vi "TLS Client.vi"() -> ()   [LabVIEW 2020, in "Test.lvlib"]
uses:
  Test.lvlib
  TCP Comms/TinyTCP.lvlib
  TCP Comms/Cert Chain.ctl
  TCP Comms/Client TLS Config.ctl
  346ab590-12ca-473f-8f0a-edbb0b931e8c.vi
  3b2e32dd-1c02-490c-a519-554a5f01b085.vi
  Server Data.ctl
  TCP Comms/State.ctl
  Client Data.ctl
panel:
  out "Error":errorcluster
  out "Server Data":T1
  in  "Client Data":T2 {"Slide" scale=0.0..10.0}
  in  "Close":bool
  in  "Open":bool
  out "Client State":T3
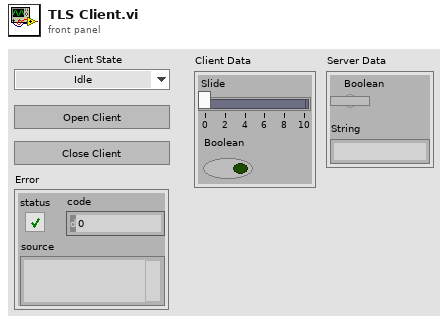
[diagram p1: front panel]
types:
  T1 = typedef "Test.lvlib/Server Data.ctl" = cluster{"Boolean":bool, "String":string}
  T2 = typedef "Test.lvlib/Client Data.ctl" = cluster{"Slide":dbl, "Boolean":bool}
  T3 = typedef "TinyTCP.lvlib/State.ctl" = enum16{"Idle", "Starting", "Connecting", "Connected", "Disconnecting", "Stopped"}
  T4 = typedef "TinyTCP.lvlib/Cert Chain.ctl" = cluster{"Path":path, "Format":enum32{"X.509 (PEM)"}}
  T5 = typedef "TinyTCP.lvlib/Client TLS Config.ctl" = cluster{"Use OS Certificates":bool, "Cert Chains":T4[], "Server Cert Name":string}
  T6 = typedef "TinyTCP.lvlib/Instance.ctl" = refnum<data-value>
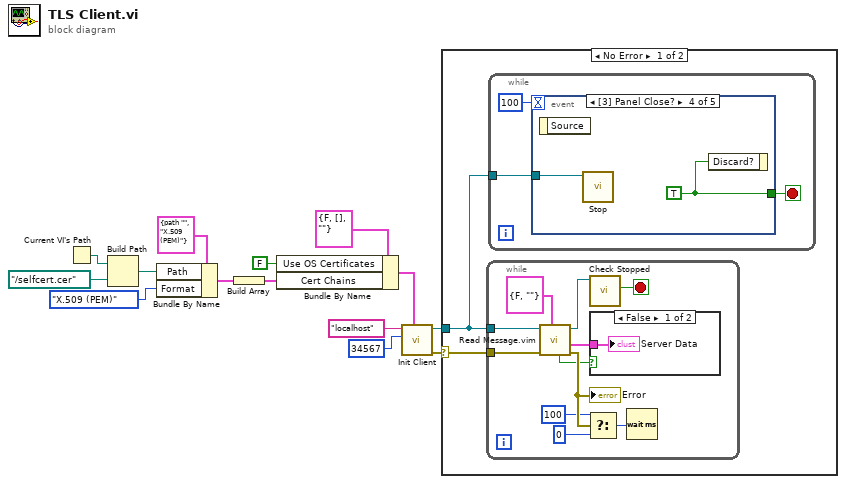
[diagram p0: block diagram]
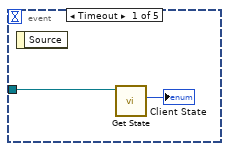
[diagram p3: hidden frame]
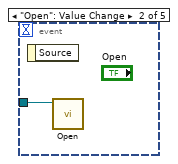
[diagram p4: hidden frame]
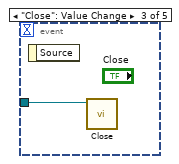
[diagram p5: hidden frame]
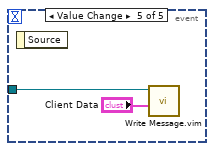
[diagram p6: hidden frame]
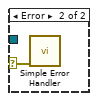
[diagram p7: hidden frame]
diagram:
  n1 = Current VI's Path() -> (path=w10:path)
  n2 = Build Path(base path=w10, name or relative path=path "../selfcert.cer") -> (appended path=w8:path)
  n3 = Bundle By Name(cluster=T4 {"Path"=path "", "Format"=enum."X.509 (PEM)"} ("Cert Chain"), "Path"=w8, "Format"=enum32{"X.509 (PEM)"}."X.509 (PEM)") -> (w6:T4)
  n4 = Build Array(w6) -> (w5:T4[])
  n5 = Bundle By Name(cluster=T5 {"Use OS Certificates"=FALSE, "Cert Chains"=[], "Server Cert Name"=""} ("Client TLS Config"), "Use OS Certificates"=FALSE, "Cert Chains"=w5) -> (w13:T5)
  n6 = call "Init Client.vi"("Client TLS Config (Disabled)"=w13, "Port"=u16 34567, "Host"="localhost") -> ("error out"=w2:errorcluster, "TinyTCP Client"=w1:T6)  [unwired: 7 in]
  n7 = case shown="No Error" w2 {
    selector: w2 -> [w16 w40]
    tunnel: w1 -> [w15 _]
    frame No Error {
      n8 = while {
        tunnel: w15 -> [w26]
        tunnel: w16 -> [w25]
        stop <- w18 stop-if-true
        n9 = call "Read Message.vim"("Data Type (String)"=T1 {"Boolean"=FALSE, "String"=""} ("Server Data"), "error in (no error)"=w25, "TCP Comm In"=w26) -> ("error out"=w27:errorcluster, "Data"=w23:T1, "TCP Comm"=w19:T6, "Timeout?"=w17:bool)  [unwired: 3 in, 2 out]
        "Error" <- w27
        n10 = Select(t=u32 100, s=w27, f=u32 0 ("milliseconds to wait")) -> (s? t:f=w21:u32)
        n11 = call "Check Stopped.vi"("TCP Comm In"=w19) -> ("Stopped?"=w18:bool)  [unwired: 9 in, 1 out]
        n12 = case shown="False" w17 {
          tunnel: w23 -> [w28 _]
          frame False {
            "Server Data" <- w28
          }
          frame True {
          }
        }
        n13 = Wait (ms)(milliseconds to wait=w21) -> ()  [unwired: 1 out]
      }
      n14 = while {
        tunnel: w15 -> [w31]
        stop <- w30 stop-if-true
        n15 = event shown="[3] Panel Close?" {
          selector: _ -> [_ _ _ _ _]
          dyn-events: _ -> [_ _ _ _ _]
          timeout: 100 -> [_ _ _ _ _]
          tunnel: w31 -> [w33 w34 w35 w37 w39]
          tunnel: [_ _ _ w36 _] -> w30
          event Timeout {
            n16 = event-data() -> ()  [unwired: 1 in, 1 out]
            n17 = call "Get State.vi"("TCP Comm In"=w33) -> ("State"=→"Client State":T3)  [unwired: 9 in, 1 out]
          }
          event "Open": Value Change {
            n18 = event-data() -> ()  [unwired: 1 in, 1 out]
            n19 = call "Open.vi"("TCP Comm"=w34) -> ()  [unwired: 10 in, 1 out]
          }
          event "Close": Value Change {
            n20 = event-data() -> ()  [unwired: 1 in, 1 out]
            n21 = call "Close.vi"("TCP Comm"=w35) -> ()  [unwired: 10 in, 1 out]
          }
          event Panel Close? {
            w36 = TRUE
            n22 = event-data() -> ()  [unwired: 1 in, 1 out]
            n23 = call "Stop.vi"("TCP Comm"=w37) -> ()  [unwired: 10 in, 1 out]
            n24 = event-data("Discard?"=w36) -> ()  [unwired: 1 in, 1 out]
          }
          event Value Change {
            n25 = event-data() -> ()  [unwired: 1 in, 1 out]
            n26 = call "Write Message.vim"("Data"="Client Data", "TCP Comm In"=w39) -> ()  [unwired: 7 in, 3 out]
          }
        }
      }
    }
    frame Error {
      n27 = call <vilib>:"Simple Error Handler.vi"("error in (no error)"=w40) -> ()  [unwired: 4 in, 5 out]
    }
  }
